vi "IndexVelocity_Write.vi"(0 "Axis In":T2, 5 "Index (0)":T1, 7 "Velocity":dbl, 11 "error in (no error)":errorcluster) -> (4 "Axis Out":T2, 6 "Index (duplicate)":T1, 15 "error out":errorcluster)   [LabVIEW 2009]
uses:
  typedefs/AxisSelect_Enum.ctl
  typedefs/Ultra3000/Index_Numeric.ctl
  typedefs/Ultra3000/Cmds.ctl
  typedefs/Ultra3000/Func.ctl
  globals/AxisSpace.vi
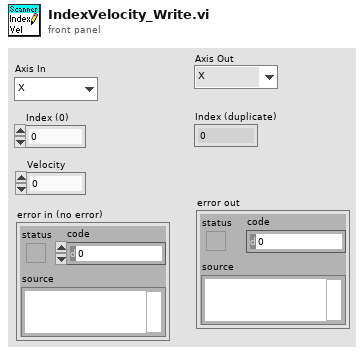
[diagram p1: front panel]
types:
  T1 = typedef "Index_Numeric.ctl" = u8
  T2 = typedef "AxisSelect_Enum.ctl" = enum16{"X", "Y", "Z", "Axis Space"}
  T3 = typedef "Func.ctl" = u16
  T4 = typedef "Cmds.ctl" = u16
  T5 = typedef "AxisSpaceCfg.ctl" = T6[]
  T6 = typedef "AxisCfg.ctl" = cluster{"Addr":u8, "Conv Factor":dbl, "Forward Limit":dbl, "Reverse Limit":dbl, "Enable Limits":bool}
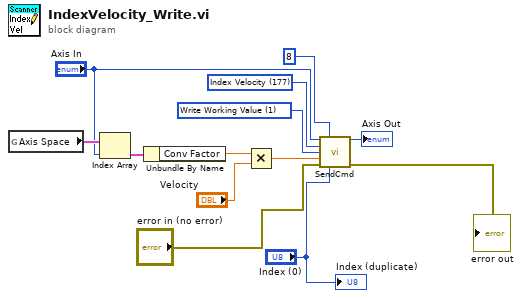
[diagram p0: block diagram]
diagram:
  w12 = T3 1 items=["Read Working Value", "Write Working Value", "Read Non-Volatile Value", "Write Non-Volatile and Woring Value", "Copy Non-Volatile Value to Working Value", "Copy Working Value to Non-Volatile Value", "Read Default Value", "Copy Default Value to Non-Volatile and Working Values", "Read Min Value", "Read Max Value", "Read Array Index Min", "Read Array Index Max"] ("Function")
  w13 = T4 177 items=["Position Command"=128, "Run Status"=117, "Fault Status"=116, "Position Error"=129, "Auto-Start Homing"=196, "Start Homing"=205, "Homing Type"=197, "Motor Position"=126, "Velocity Motor"=133, "Power-Up Status"=1, "Drive Name"=6, "Position Window Size"=22, "Position Window Time"=23, "Zero Speed Limit"=34, "Speed Window Size"=35, "Up to Speed Limit"=37, "Forward Current Limit"=47, "Reverse Current Limit"=48, "Override Mode"=67, "Operation Mode"=90, "Host Control Mode"=97, "Reset Drive"=106, "Drive Enable"=107, "Setpoint Current"=108, "Setpoint Velocity"=109, "Setpoint Acceleration"=110, "Reset Faults"=111, "Position Comparator"=349, "Postition Comparator Polarity"=350, "Position Rollover Enable"=404, "Baud Rate"=80, "Frame Format"=81, "Drive Address"=82, "Broadcast Address"=83, "Auto-start Indexing"=88, "Start Index"=112, "Host Index"=184, "Index Type"=174, "Index Dist/Pos"=175, "Index Reg Dist"=176, "Index Velocity"=177, "Index Acceleration"=178, "Index Deceleration"=179, "Index Dwell"=180, "Index Count"=181, "Index Termination"=182, "Index Pointer"=183, "Index Abort Deceleration"=185, "Positive Soft Pos Limit"=216, "Define Home"=113, "Negative Soft Pos Limit"=217] ("Command")
  n1 = global read "AxisSpace.vi" "Axis Space"() -> (w9:T5)
  n2 = Index Array(array=w9, index="Axis In") -> (element=w7:T6)
  n3 = Unbundle By Name(w7) -> ("Conv Factor"=w6:dbl)
  n4 = Multiply(x=w6, y="Velocity") -> (x*y=w4:dbl)
  n5 = call "SendCmd.vi"("Axis In"="Axis In", "Data Length Constant (0)"=u8 8, "Command"=w13, "Function"=w12, "Data (0)"=w4, "error in (no error)"="error in (no error)", "Index (0)"="Index (0)") -> ("Axis Out"=→"Axis Out":T2, "error out"=→"error out":errorcluster)  [unwired: 5 in, 2 out]
  "Index (duplicate)" <- "Index (0)"
